vi "SetTension.vi"(7 "command":enum16{"Move", "Tension"}(ring), 8 "error in (no error)":errorcluster, 11 "Tapedrive_ESP301 in":refnum<class "Tapedrive_ESP301.lvclass">) -> (0 "error out":errorcluster, 3 "Tapedrive_ESP301 out":refnum<class "Tapedrive_ESP301.lvclass">)   [LabVIEW 2013, in "Tapedrive_ESP301.lvclass"]
uses:
  Tapedrive_ESP301.lvclass
  shared/OnOffTypeDef.ctl
panel:
  out "Settings.Decceleration":T1
  out "Settings.Acceleration":T1
  out "Settings.Velocity":T1
  out "spreadsheet string":string
  out "settings needed":bool
  out "Error Message":string
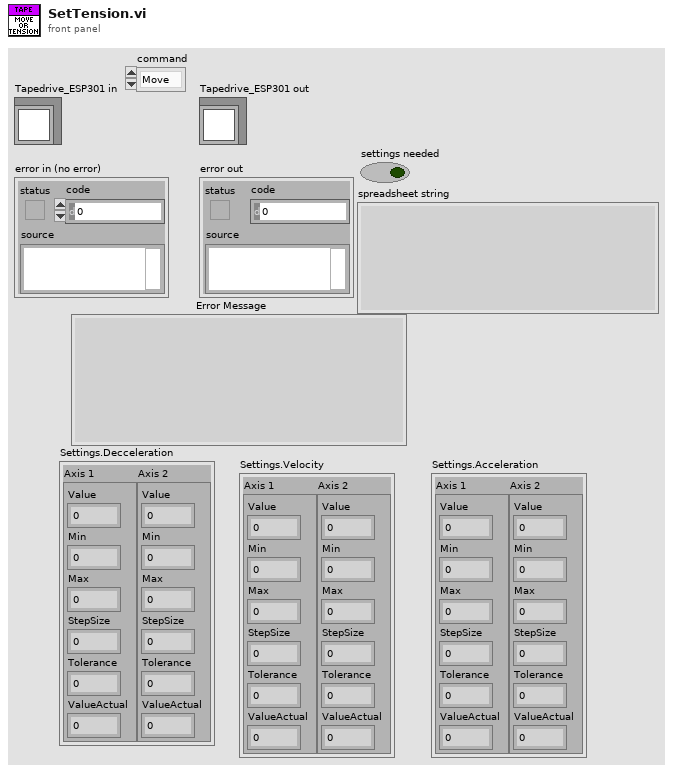
[diagram p1: front panel]
types:
  T1 = cluster{"Axis 1":cluster{"Value":dbl, "Min":dbl, "Max":dbl, "StepSize":dbl, "Tolerance":dbl, "ValueActual":dbl}, "Axis 2":cluster{"Value":dbl, "Min":dbl, "Max":dbl, "StepSize":dbl, "Tolerance":dbl, "ValueActual":dbl}}
  T2 = typedef "OnOffTypeDef.ctl" = enum16{"off", "on"}
  T3 = typedef "Direction.ctl" = enum16{"Forward", "Backward", "Undefined"}
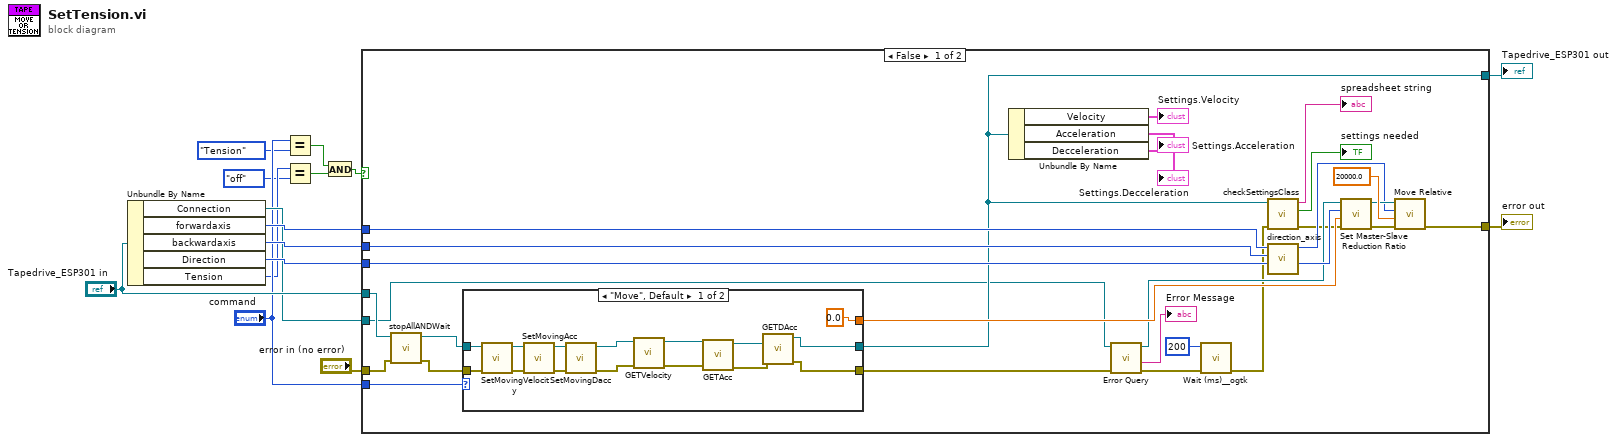
[diagram p0: block diagram]
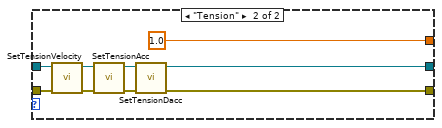
[diagram p2: hidden frame]
diagram:
  n1 = Unbundle By Name("Tapedrive_ESP301 in") -> ("Connection"=w10:refnum<visa-resource-name>, "forwardaxis"=w13:i16, "backwardaxis"=w12:i16, "Direction"=w11:T3, "Tension"=w7:T2)
  n2 = Equal?(x="command", y=enum16{"Move", "Tension"}."Tension") -> (x = y?=w5:bool)
  n3 = Equal?(x=w7, y=OnOffTypeDef."off") -> (x = y?=w4:bool)
  n4 = And(x=w5, y=w4) -> (x .and. y?=w2:bool)
  n5 = case shown="False" w2 {
    tunnel: [w44 w69] -> w15
    tunnel: "Tapedrive_ESP301 in" -> [w20 w70]
    tunnel: w13 -> [w43 _]
    tunnel: w12 -> [w42 _]
    tunnel: w11 -> [w41 _]
    tunnel: w10 -> [w16 _]
    tunnel: "command" -> [w37 _]
    tunnel: [w24 w70] -> w3
    tunnel: "error in (no error)" -> [w18 w69]
    frame False {
      n6 = call "stopAllANDWait.vi"("error in (no error)"=w18, "Tapedrive_ESP301 in"=w20) -> ("error out"=w17:errorcluster, "Tapedrive_ESP301 out"=w19:refnum<class "Tapedrive_ESP301.lvclass">)  [unwired: 8 in]
      n7 = case shown="\"Move\", Default" w37 {
        tunnel: [w49 w68] -> w24
        tunnel: w19 -> [w56 w63]
        tunnel: w17 -> [w57 w62]
        tunnel: [w45 w61] -> w34
        tunnel: [0.0 ("Reduction Ratio (0)") 1.0 ("Reduction Ratio (0)")] -> w36
        frame "Move", Default {
          n8 = call "SetMovingVelocity.vi"("error in (no error)"=w57, "Tapedrive_ESP301 in"=w56) -> ("error out"=w58:errorcluster, "Tapedrive_ESP301 out"=w59:refnum<class "Tapedrive_ESP301.lvclass">)  [unwired: 8 in]
          n9 = call "SetMovingAcc.vi"("error in (no error)"=w58, "Tapedrive_ESP301 in"=w59) -> ("error out"=w53:errorcluster, "Tapedrive_ESP301 out"=w54:refnum<class "Tapedrive_ESP301.lvclass">)  [unwired: 8 in]
          n10 = call "SetMovingDacc.vi"("error in (no error)"=w53, "Tapedrive_ESP301 in"=w54) -> ("error out"=w48:errorcluster, "Tapedrive_ESP301 out"=w52:refnum<class "Tapedrive_ESP301.lvclass">)  [unwired: 8 in]
          n11 = call "GETVelocity.vi"("error in (no error)"=w48, "Tapedrive_ESP301 in"=w52) -> ("error out"=w47:errorcluster, "Tapedrive_ESP301 out"=w51:refnum<class "Tapedrive_ESP301.lvclass">)  [unwired: 8 in]
          n12 = call "GETAcc.vi"("error in (no error)"=w47, "Tapedrive_ESP301 in"=w51) -> ("error out"=w46:errorcluster, "Tapedrive_ESP301 out"=w50:refnum<class "Tapedrive_ESP301.lvclass">)  [unwired: 8 in]
          n13 = call "GETDAcc.vi"("error in (no error)"=w46, "Tapedrive_ESP301 in"=w50) -> ("error out"=w45:errorcluster, "Tapedrive_ESP301 out"=w49:refnum<class "Tapedrive_ESP301.lvclass">)  [unwired: 8 in]
        }
        frame "Tension" {
          n14 = call "SetTensionVelocity.vi"("error in (no error)"=w62, "Tapedrive_ESP301 in"=w63) -> ("error out"=w65:errorcluster, "Tapedrive_ESP301 out"=w64:refnum<class "Tapedrive_ESP301.lvclass">)  [unwired: 8 in]
          n15 = call "SetTensionAcc.vi"("error in (no error)"=w65, "Tapedrive_ESP301 in"=w64) -> ("error out"=w66:errorcluster, "Tapedrive_ESP301 out"=w67:refnum<class "Tapedrive_ESP301.lvclass">)  [unwired: 8 in]
          n16 = call "SetTensionDacc.vi"("error in (no error)"=w66, "Tapedrive_ESP301 in"=w67) -> ("error out"=w61:errorcluster, "Tapedrive_ESP301 out"=w68:refnum<class "Tapedrive_ESP301.lvclass">)  [unwired: 8 in]
        }
      }
      n17 = Unbundle By Name(w24) -> ("Velocity"=→"Settings.Velocity":T1, "Acceleration"=→"Settings.Acceleration":T1, "Decceleration"=→"Settings.Decceleration":T1)
      n18 = call <instrlib>:"Error Query.vi"("error in (no error)"=w34, "VISA resource name"=w16) -> ("error out"=w30:errorcluster, "Error Message"=→"Error Message":string, "VISA resource name out"=w33:refnum<visa-resource-name>)  [unwired: 3 out]
      n19 = call <userlib>:"Wait (ms)__ogtk.vi"("error in (no error)"=w30, "milliseconds to wait"=u32 200) -> ("error out"=w28:errorcluster)  [unwired: 8 in, 1 out]
      n20 = call "checkSettingsClass.vi"("error in (no error)"=w28, "Tapedrive_ESP301 in"=w24) -> ("error in (no error) 2"=w27:errorcluster, "settings needed"=→"settings needed":bool, "spreadsheet string"=→"spreadsheet string":string)  [unwired: 5 in, 2 out]
      n21 = call "direction_axis.vi"("Direction"=w41, "backwardaxis"=w42, "forwardaxis"=w43) -> ("Slave"=w35:i16, "Master"=w31:i16)  [unwired: 7 in]
      n22 = call <instrlib>:"Set Master-Slave Reduction Ratio.vi"("error in (no error)"=w27, "Reduction Ratio (0)"=w36, "Axis (1)"=w35, "VISA resource name"=w33) -> ("error out"=w38:errorcluster, "VISA resource name out"=w39:refnum<visa-resource-name>)  [unwired: 2 in]
      n23 = call <instrlib>:"Move Relative.vi"("error in (no error)"=w38, "Position (0 units)"=20000.0, "Axis (1)"=w31, "VISA resource name"=w39) -> ("error out"=w44:errorcluster)  [unwired: 2 in, 1 out]
    }
    frame True {
    }
  }
  "error out" <- w15
  "Tapedrive_ESP301 out" <- w3
